vi "Time.Delta Time Secs.vi"(11 "Start":dbl) -> (2 "Dur_Sec_Str":string, 3 "Dur(s)":dbl)   [LabVIEW 2019]
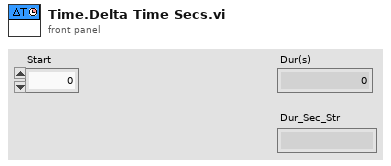
[diagram p1: front panel]
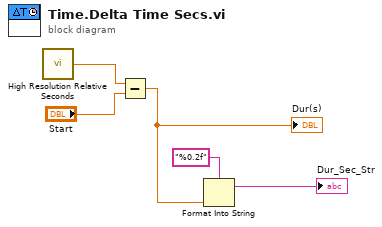
[diagram p0: block diagram]
diagram:
  n1 = call <vilib>:"High Resolution Relative Seconds.vi"() -> ("relative seconds"=w5:dbl)
  n2 = Subtract(x=w5, y="Start") -> (x-y=w3:dbl)
  "Dur(s)" <- w3
  n3 = Format Into String(format string="%0.2f", w3) -> (resulting string=→"Dur_Sec_Str":string)  [unwired: 2 in, 1 out]
